vi "emptyProcess.vi"(11 "ID":u32=1336) -> (0 "return":dbl=87.0, 1 "ProcessWorkingSetSize min":i32=204800, 2 "ProcessWorkingSetSize max":i32=1413120)   [LabVIEW 2016]
uses:
  processHandles.dll
panel:
  in  "min":i32
  in  "max":i32
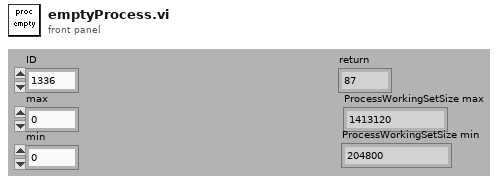
[diagram p1: front panel]
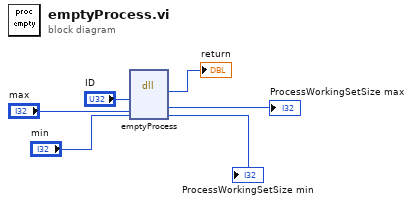
[diagram p0: block diagram]
diagram:
  n1 = dll-call lib="C:/Technology Lab/NI-2010/Trunk/Utility/Project Memory Manager/Project Manager/processHandles.dll" fn="emptyProcess"("ID"="ID", "max"="max", "min"="min") -> ("return type"=→"return":i32, "max"=→"ProcessWorkingSetSize max":i32, "min"=→"ProcessWorkingSetSize min":i32)  [unwired: 4 in, 2 out]
